vi "Get SMO Public API.vi"(8 "error in (no error)":errorcluster, 11 "Inst.Attocube-3DR in":refnum<class "Inst.Attocube-3DR.lvclass">) -> (0 "error out":errorcluster, 2 "Commands":string[](array[string]), 3 "Inst.Attocube-3DR out":refnum<class "Inst.Attocube-3DR.lvclass">)   [LabVIEW 2019, in "Inst.Attocube-3DR.lvclass"]
uses:
  Inst.Attocube-3DR.lvclass
  Typedefs/Inst.Attocube-3DR.Commands--Enum.ctl
  323bdc6f-b15f-4066-b5b7-bebf587f1bf8.vi
  <vilib>/Utility/Data Type/Get Type Information.vi
  <vilib>/Utility/Data Type/Get Numeric Information.vi
  <userlib>/_OpenG.lib/lvdata/lvdata.llb/Unwrap VVariant__ogtk.vi
  <userlib>/LevyLab/Instrument Framework/Instrument/Instrument.lvclass
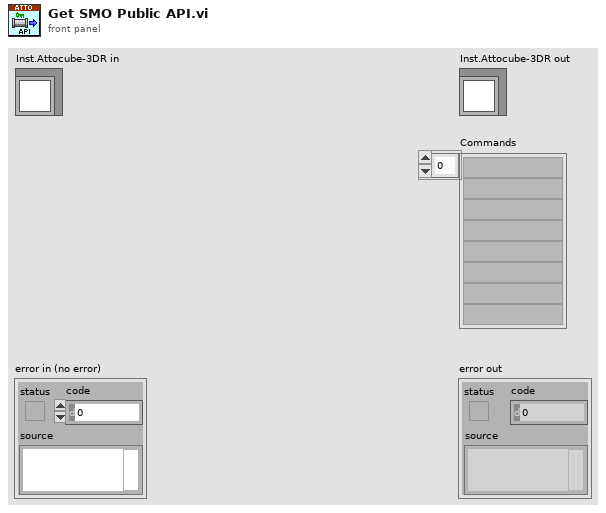
[diagram p1: front panel]
types:
  T1 = typedef "Inst.Attocube-3DR.lvclass/Inst.Attocube-3DR.Commands--Enum.ctl" = enum16{"GetStepWidth", "GetRotCount", "GetPosition", "GetSpeed", "GetStatus"}
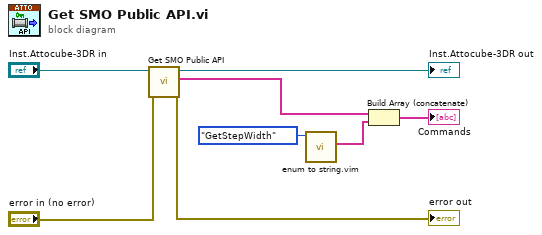
[diagram p0: block diagram]
diagram:
  n1 = call-parent "Get SMO Public API.vi"("error in (no error)"="error in (no error)", "Instrument in"="Inst.Attocube-3DR in") -> ("error out"=→"error out":errorcluster, "commands"=w8:string[], "Instrument out"=→"Inst.Attocube-3DR out":refnum<class "Inst.Attocube-3DR.lvclass">)  [unwired: 7 in]
  n2 = call "enum to string.vim"("enum in"=Inst.Attocube-3DR.Commands--Enum."GetStepWidth" ("Commands")) -> ("strings out"=w3:string[])  [unwired: 9 in, 1 out]
  n3 = Build Array (concatenate)(w8, w3) -> (→"Commands":string[])
